vi "ULx Create Channel (CompI-Counter Input-Count Edges).vi"(0 "task in":refnum<k24>, 1 "initial count":u32, 2 "count direction":i32(ring) items=["CountUp", "CountDown"], 3 "edge":i32(ring) items=["Rising", "Falling"], 5 "counters":refnum<k21>, 11 "error in":errorcluster) -> (4 "task out":refnum<k24>, 15 "error out":errorcluster)   [LabVIEW 2020]
doc: "Creates channel(s) to count the number of falling and rising edges of digital signals."
uses:
  C:/Users/William/Documents/LV 2020 builds/LeaktestDAQ/Source-v33/ULx_LV.dll
  ULx_LV.dll
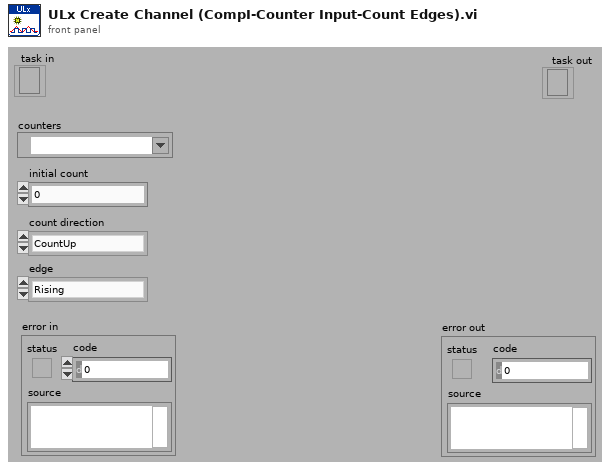
[diagram p1: front panel]
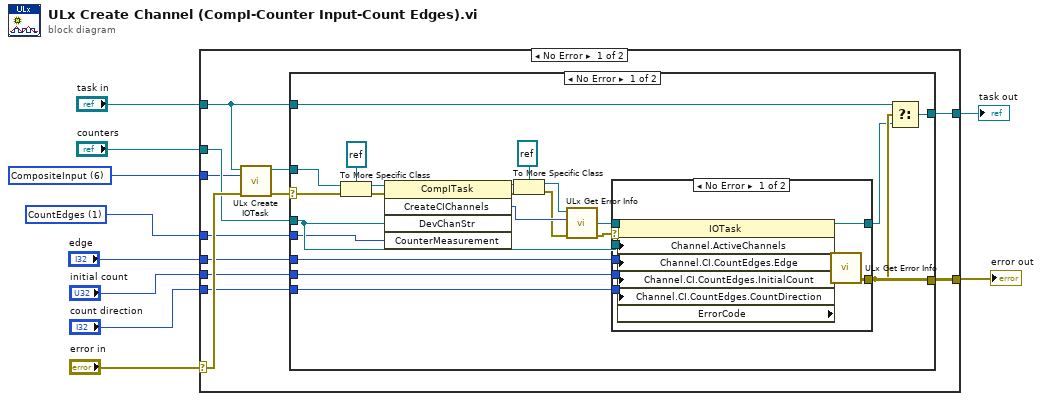
[diagram p0: block diagram]
diagram:
  w2 = 1 items=["CountEdges"=1, "Encoder"=2, "Frequency"=3, "Period"=4] ("CounterMeasurement")
  w6 = 6 items=["AnalogInput", "AnalogOutput", "DigitalInput", "DigitalOutput", "CounterInput", "CounterOutput", "CompositeInput", "CompositeOutput", "TemperatureInput"] ("taskType")
  n1 = case shown="No Error" "error in" {
    selector: "error in" -> [w22 w59]
    tunnel: "task in" -> [w11 w58]
    tunnel: "counters" -> [w17 _]
    tunnel: [w20 w58] -> w8
    tunnel: [w19 w59] -> w7
    tunnel: w6 -> [w16 _]
    tunnel: "edge" -> [w15 _]
    tunnel: "initial count" -> [w14 _]
    tunnel: "count direction" -> [w13 _]
    tunnel: w2 -> [w12 _]
    frame No Error {
      n2 = call "ULx Create IOTask.vi"("error in"=w22, "taskType"=w16, "i/o task in"=w11) -> ("error out"=w21:errorcluster, "i/o task out"=w18:refnum<k24>)  [unwired: 7 in]
      n3 = case shown="No Error" w21 {
        selector: w21 -> [w42 w57]
        tunnel: [w25 w57] -> w19
        tunnel: [w26 w56] -> w20
        tunnel: w18 -> [w40 _]
        tunnel: w17 -> [w37 _]
        tunnel: w15 -> [w33 _]
        tunnel: w14 -> [w36 _]
        tunnel: w13 -> [w35 _]
        tunnel: w12 -> [w34 _]
        tunnel: w11 -> [w27 w56]
        frame No Error {
          n4 = To More Specific Class(target class=refnum<k24> refnum, reference=w40, error in=w42) -> (specific class reference=w43:refnum<k24>, error out=w41:errorcluster)
          n5 = invoke class="CompITask" method="CreateCIChannels"(reference=w43, error in=w41, "DevChanStr"=w37, "CounterMeasurement"=w34) -> (reference out=w31:refnum<k24>, error out=w30:errorcluster, "CreateCIChannels"=w39:i32)  [unwired: 1 in, 2 out]
          n6 = To More Specific Class(target class=refnum<k24> refnum, reference=w31, error in=w30) -> (specific class reference=w28:refnum<k24>, error out=w29:errorcluster)
          n7 = call "ULx Get Error Info.vi"("error in"=w29, "ErrorCode"=w39, "task in"=w28) -> ("error out"=w38:errorcluster)  [unwired: 8 in]
          n8 = case shown="No Error" w38 {
            selector: w38 -> [w53 w55]
            tunnel: w28 -> [w52 w54]
            tunnel: w33 -> [w51 _]
            tunnel: w37 -> [w50 _]
            tunnel: [w47 w55] -> w25
            tunnel: w36 -> [w46 _]
            tunnel: w35 -> [w45 _]
            tunnel: [w44 w54] -> w24
            frame No Error {
              n9 = property class="IOTask"(reference=w52, error in=w53, "Channel.ActiveChannels"=w50, "Channel.CI.CountEdges.Edge"=w51, "Channel.CI.CountEdges.InitialCount"=w46, "Channel.CI.CountEdges.CountDirection"=w45) -> (reference out=w44:refnum<k24>, error out=w48:errorcluster, "ErrorCode"=w49:i32)
              n10 = call "ULx Get Error Info.vi"("error in"=w48, "ErrorCode"=w49, "task in"=w44) -> ("error out"=w47:errorcluster)  [unwired: 8 in]
            }
            frame Error {
            }
          }
          n11 = Select(t=w27, s=w25, f=w24) -> (s? t:f=w26:refnum<k24>)
        }
        frame Error {
        }
      }
    }
    frame Error {
    }
  }
  "error out" <- w7
  "task out" <- w8
